vi "Facade.vi"(0 "Data In":T4, 2 "Display State In":T2, 3 "Container State":T3) -> (6 "Data Out":T4, 7 "Display State Out":T2, 8 "Action":T1)   [LabVIEW 2020, in "Trigger.xctl"]
uses:
  Trigger.xctl
  <vilib>/_xctls/Action.ctl
  <vilib>/_xctls/XControlSupport.lvlib
  <vilib>/_xctls/Container State.ctl
  Data.ctl
  State.ctl
panel:
  out "context dependent":bool
  in  "Expr":string
  in  "When":u16(ring)
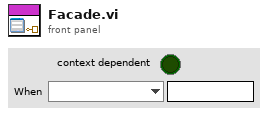
[diagram p1: front panel]
types:
  T1 = typedef "XControlSupport.lvlib/Action.ctl" = cluster{"Data Changed?":bool, "State Changed?":bool, "Action Name":string}
  T2 = typedef "Trigger.xctl/State.ctl" = cluster{"Name":string, "Strings and Formats":cluster{"Items":string[], "Formats":string[]}}
  T3 = typedef "XControlSupport.lvlib/Container State.ctl" = cluster{"Indicator?":bool, "Run Mode?":bool, " Refnum":refnum<vi>}
  T4 = typedef "Trigger.xctl/Data.ctl" = cluster{"When":string, "Expr":string}
  T5 = typedef "LVPoint32TypeDef.ctl" = cluster{"Horizontal":i32, "Vertical":i32}
  T6 = typedef "LVRectTypeDef.ctl" = cluster{"Left":i16, "Top":i16, "Right":i16, "Bottom":i16}
  T7 = typedef "LVPositionTypeDef.ctl" = cluster{"Left":i32, "Top":i32}
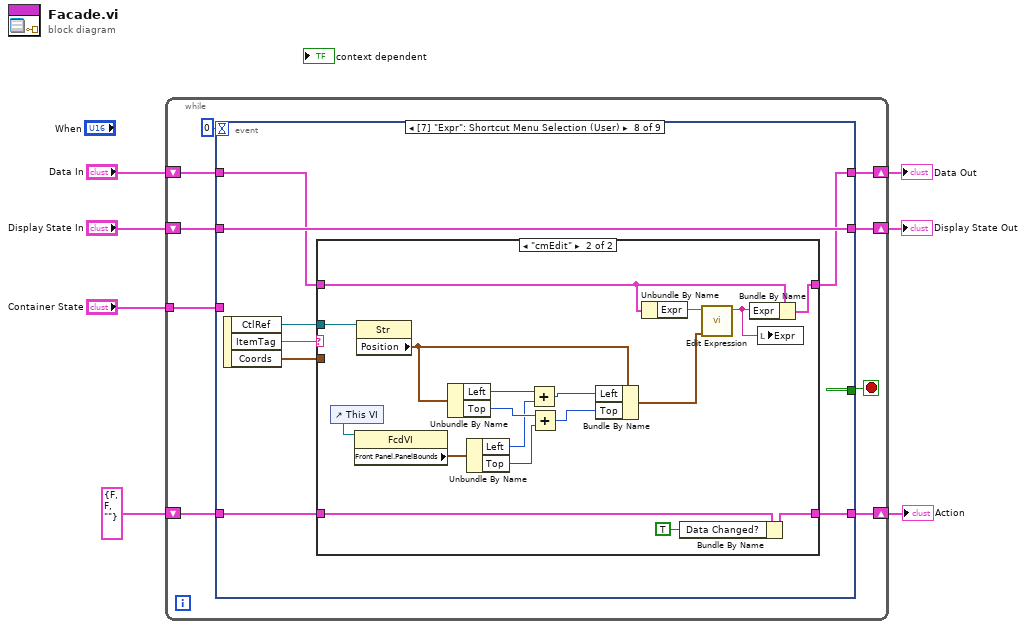
[diagram p0: block diagram]
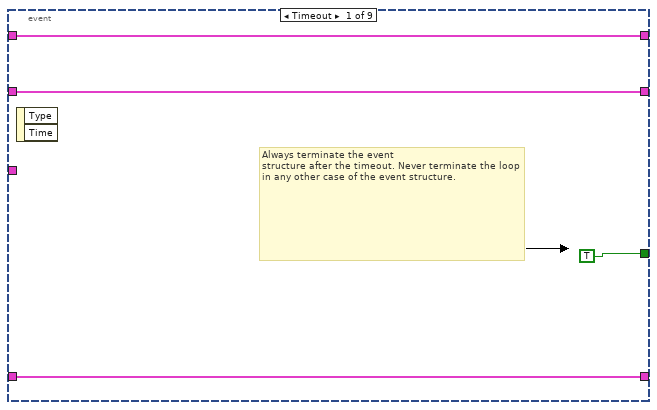
[diagram p2: hidden frame]
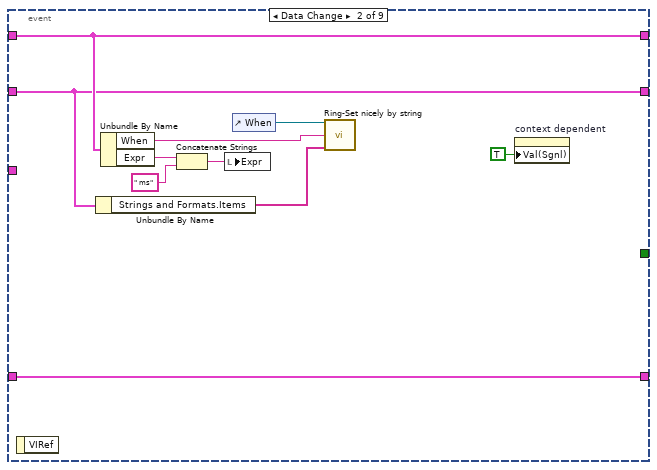
[diagram p3: hidden frame]
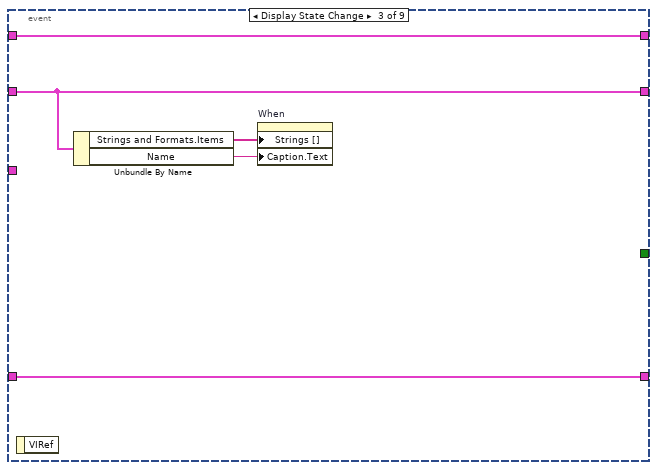
[diagram p4: hidden frame]
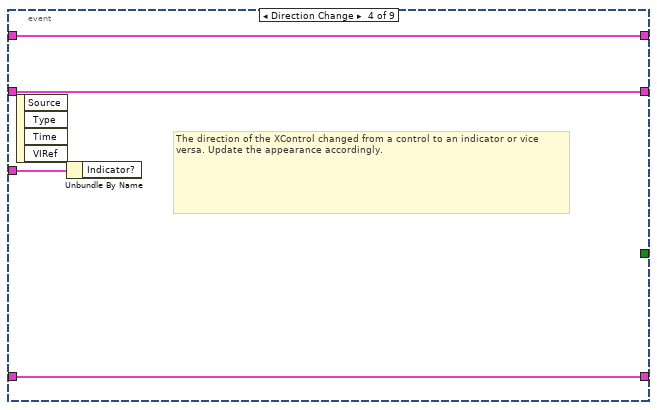
[diagram p5: hidden frame]
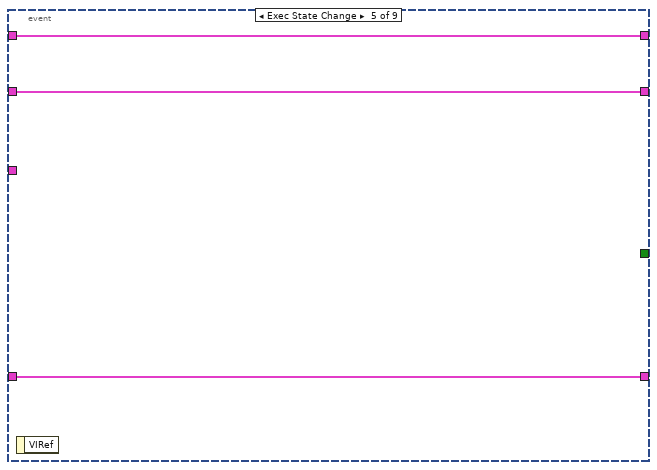
[diagram p6: hidden frame]
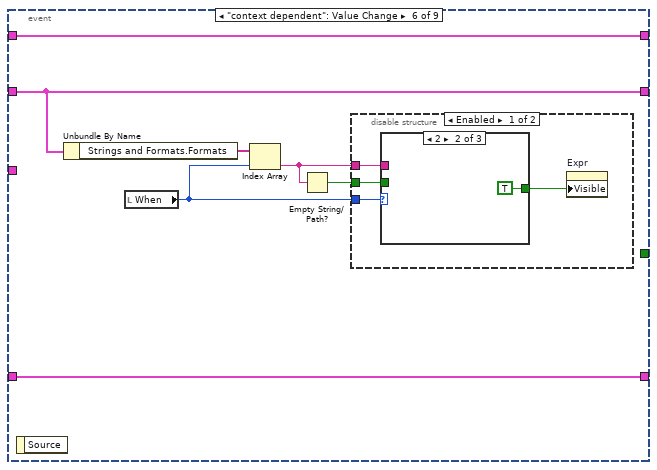
[diagram p7: hidden frame]
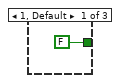
[diagram p8: hidden frame]
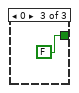
[diagram p9: hidden frame]
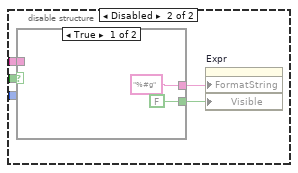
[diagram p10: hidden frame]
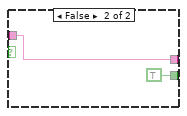
[diagram p11: hidden frame]
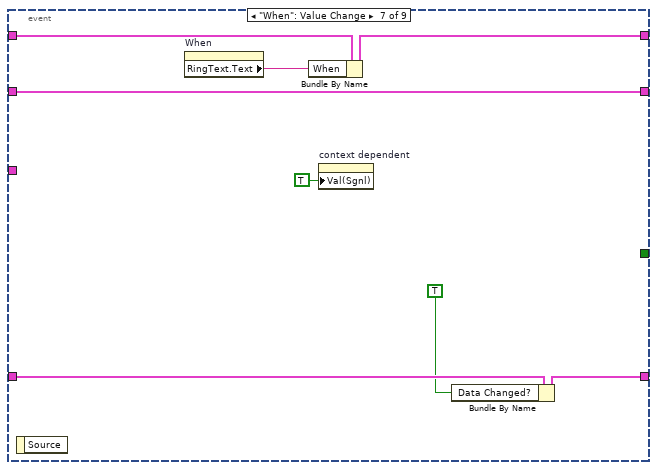
[diagram p12: hidden frame]
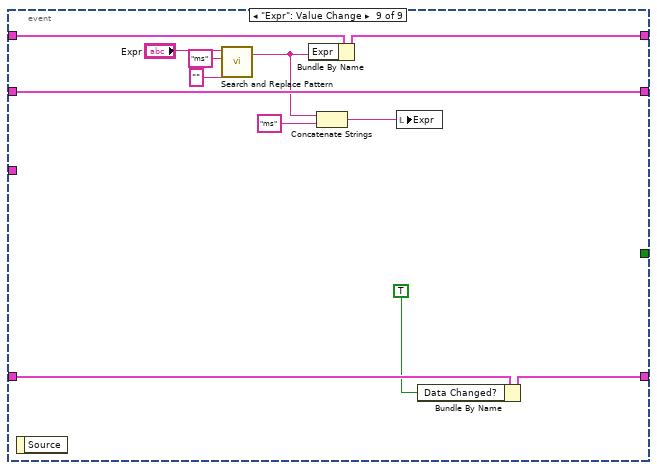
[diagram p14: hidden frame]
diagram:
  n1 = while {
    shift-right: [w15] -> w4
    shift-left: "Display State In" -> [w16]
    tunnel: "Container State" -> [w12]
    shift-right: [w10] -> w7
    shift-left: "Data In" -> [w11]
    shift-right: [w8] -> w2
    shift-left: T1 {"Data Changed?"=FALSE, "State Changed?"=FALSE, "Action Name"=""} ("Action") -> [w9]
    stop <- w14 stop-if-true
    n2 = event shown="[7] \"Expr\": Shortcut Menu Selection (User)" {
      selector: _ -> [_ _ _ _ _ _ _ _ _]
      dyn-events: _ -> [_ _ _ _ _ _ _ _ _]
      timeout: 0 -> [_ _ _ _ _ _ _ _ _]
      tunnel: w16 -> [w18 w26 w33 w38 w42 w47 w72 w80 w112]
      tunnel: [w18 w26 w33 w38 w42 w47 w72 w80 w112] -> w15
      tunnel: [TRUE _ _ _ _ _ _ _ _] -> w14
      tunnel: w12 -> [_ _ _ w39 _ _ _ _ _]
      tunnel: w11 -> [w17 w29 w35 w37 w41 w49 w71 w78 w111]
      tunnel: [w17 w29 w35 w37 w41 w49 w69 w77 w109] -> w10
      tunnel: [w19 w30 w34 w36 w40 w48 w66 w73 w108] -> w8
      tunnel: w9 -> [w19 w30 w34 w36 w40 w48 w70 w74 w110]
      event Timeout {
        # "Always terminate the event\nstructure after the timeout. Never terminate the loop in any other case of the event structure."
        n3 = event-data() -> ()  [unwired: 1 in, 2 out]
      }
      event Data Change {
        n4 = event-data() -> ()  [unwired: 1 in, 1 out]
        n5 = Unbundle By Name(w26) -> ("Strings and Formats.Items"=w25:string[])
        n6 = Unbundle By Name(w29) -> ("When"=w24:string, "Expr"=w23:string)
        n7 = Concatenate Strings(w23, " ms" ("string")) -> (w22:string)
        n8 = local write "Expr"(w22) -> ()
        n9 = control-ref of="When"() -> (w27:refnum<vi>)
        n10 = call "Ring-Set nicely by string.vi"("Ring in"=w27, "Device"=w24, "Strings []"=w25) -> ()  [unwired: 8 in, 5 out]
        n11 = property on="context dependent" class="Bool (strict)"("Val(Sgnl)"=TRUE ("Value (Signaling)")) -> ()  [unwired: 2 in, 2 out]
      }
      event Display State Change {
        n12 = event-data() -> ()  [unwired: 1 in, 1 out]
        n13 = Unbundle By Name(w33) -> ("Strings and Formats.Items"=w32:string[], "Name"=w31:string)
        n14 = property on="When" class="Ring (strict)"("Strings []"=w32, "Caption.Text"=w31) -> ()  [unwired: 2 in, 2 out]
      }
      event Direction Change {
        # "The direction of the XControl changed from a control to an indicator or vice versa. Update the appearance accordingly."
        n15 = event-data() -> ()  [unwired: 1 in, 4 out]
        n16 = Unbundle By Name(w39) -> ()  [unwired: 1 out]
      }
      event Exec State Change {
        n17 = event-data() -> ()  [unwired: 1 in, 1 out]
      }
      event "context dependent": Value Change {
        n18 = event-data() -> ()  [unwired: 1 in, 1 out]
        n19 = Unbundle By Name(w47) -> ("Strings and Formats.Formats"=w46:string[])
        n20 = local read "When"() -> (w43:u16)
        n21 = Index Array(array=w46, index=w43) -> (element=w45:string)
        n22 = Empty String/Path?(string/path=w45) -> (empty?=w44:bool)
        n23 = disable-structure shown="Enabled" {
          disable-tunnel: w45 -> [w52 w58]
          disable-tunnel: w44 -> [w51 w57]
          disable-tunnel: w43 -> [w50 _]
          frame Enabled {
            n24 = case shown="2" w50 {
              tunnel: [FALSE TRUE FALSE] -> w53
              tunnel: w52 -> [_ _ _]
              tunnel: w51 -> [_ _ _]
              frame 1, Default {
              }
              frame 2 {
              }
              frame 0 {
              }
            }
            n25 = property on="Expr" class="Str"("Visible"=w53) -> ()  [unwired: 2 in, 2 out]
          }
          frame Disabled {
            n26 = case shown="True" w57 {
              tunnel: [FALSE TRUE] -> w60
              tunnel: ["%#g" w63] -> w59
              tunnel: w58 -> [_ w63]
              frame True {
              }
              frame False {
              }
            }
            n27 = property on="Expr" class="Str"("FormatString"=w59, "Visible"=w60) -> ()  [unwired: 2 in, 2 out]
          }
        }
      }
      event "When": Value Change {
        n28 = event-data() -> ()  [unwired: 1 in, 1 out]
        n29 = property on="When" class="Ring (strict)"() -> ("RingText.Text"=w67:string)  [unwired: 2 in, 2 out]
        n30 = Bundle By Name(cluster=w71, "When"=w67) -> (w69:T4)
        n31 = property on="context dependent" class="Bool (strict)"("Val(Sgnl)"=TRUE ("Value (Signaling)")) -> ()  [unwired: 2 in, 2 out]
        n32 = Bundle By Name(cluster=w70, "Data Changed?"=TRUE) -> (w66:T1)
      }
      event "Expr": Shortcut Menu Selection (User) {
        n33 = event-data() -> ("CtlRef"=w75:refnum<vi>, "ItemTag"=w79:string, "Coords"=w76:T5)  [unwired: 1 in]
        n34 = case shown="\"cmEdit\"" w79 {
          tunnel: w78 -> [w82 w99]
          tunnel: [w82 w98] -> w77
          tunnel: w76 -> [_ _]
          tunnel: w75 -> [_ w88]
          tunnel: w74 -> [w81 w85]
          tunnel: [w81 w84] -> w73
          frame "", Default {
          }
          frame "cmEdit" {
            n35 = control-ref of="This VI"() -> (w90:refnum<vi>)
            n36 = property class="FcdVI"(reference=w90) -> ("Front Panel.PanelBounds"=w91:T6)  [unwired: 1 in, 2 out]
            n37 = property class="Str"(reference=w88) -> ("Position"=w87:T7)  [unwired: 1 in, 2 out]
            n38 = Unbundle By Name(w87) -> ("Left"=w92:i32, "Top"=w96:i32)
            n39 = Unbundle By Name(w91) -> ("Left"=w94:i16, "Top"=w95:i16)
            n40 = Add(x=w92, y=w94) -> (x+y=w93:i32)
            n41 = Add(x=w96, y=w95) -> (x+y=w97:i32)
            n42 = Bundle By Name(cluster=w87, "Left"=w93, "Top"=w97) -> (w89:T7)
            n43 = Unbundle By Name(w99) -> ("Expr"=w100:string)
            n44 = Bundle By Name(cluster=w85, "Data Changed?"=TRUE) -> (w84:T1)
            n45 = call "Edit Expression.vi"("Coords"=w89, "Expr In"=w100) -> ("Expr Out"=w86:string)  [unwired: 9 in]
            n46 = Bundle By Name(cluster=w99, "Expr"=w86) -> (w98:T4)
            n47 = local write "Expr"(w86) -> ()
          }
        }
      }
      event "Expr": Value Change {
        n48 = event-data() -> ()  [unwired: 1 in, 1 out]
        n49 = call <vilib>:"Search and Replace Pattern.vi"("string"="Expr", "regular expression (\"\")"="ms" ("regular expression (\"\")"), "replace string (\"\")"="" ("replace string (\"\")")) -> ("result string"=w103:string)  [unwired: 2 in, 1 out]
        n50 = Bundle By Name(cluster=w111, "Expr"=w103) -> (w109:T4)
        n51 = Concatenate Strings(w103, "ms" ("regular expression (\"\")")) -> (w101:string)
        n52 = local write "Expr"(w101) -> ()
        n53 = Bundle By Name(cluster=w110, "Data Changed?"=TRUE) -> (w108:T1)
      }
    }
  }
  "Display State Out" <- w4
  "Data Out" <- w7
  "Action" <- w2
